vi "modbus slave new.vi"() -> ()   [LabVIEW 2016]
uses:
  <vilib>/NI/Modbus Library/API/Wrapper/Create TCP Slave.vi
  <vilib>/NI/Modbus Library/API/Slave/Modbus Slave.lvclass
  <vilib>/NI/Modbus Library/API/Wrapper/API Main.lvlib
  <vilib>/ptbypt/NI_PtbyPt.lvlib
panel:
  out "status":bool
  in  "写入registers to write":u16[](array[numeric])
  out "读取register values":u16[](array[numeric])
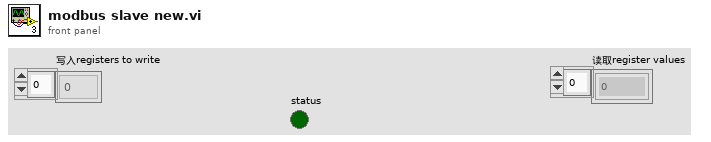
[diagram p1: front panel]
types:
  T1 = cluster{"测量量程":dbl, "测量精度":dbl, "测量间隔":dbl, "消解温度":dbl, "消解时长":dbl, "空白校准时间":timestamp, "曲线截距":dbl, "曲线斜率":dbl, "测量检出限":dbl, "测量信号值":dbl, "线性相关系数":dbl, "二次多项式系数":dbl, "标样校准时间":timestamp, "单位":u16}
  T2 = typedef "LVDateTimeRec.ctl" = cluster{"秒数的小数部分":dbl, "秒":i32, "分":i32, "时":i32, "日":i32, "月":i32, "年":i32, "天数（周）":i32, "天数（年）":i32, "DST":i32}
  T3 = enum16{"启动整机", "停止整机", "标样核查", "加标回收", "平行样测试", "零点核查", "跨度核查", "校零", "校标"}
  T4 = cluster{"status":bool, "代码":u16, "source":string}
  T5 = cluster{"系统时间":timestamp, "工作状态":enum16{"空闲", "水样测试", "标样核查", "零点核查", "跨度核查", "空白测试", "平行样测试", "加标回收", "空白校准", "标样校准", "初始化（清洗）"}, "测量模式":enum16{"待机", "连续模式", "周期模式", "定点模式", "受控模式", "手动模式"}, "告警代码":enum16{"无告警", "缺试剂告警", "缺水样告警", "缺蒸馏水告警", "缺标液告警", "仪表漏液告警", "标定异常告警", "超量程告警", "加热异常", "低试剂预警", "超上限告警", "超下限告警", "仪表内部其他异常", "滴定异常告警", "电极异常告警", "量程切换告警", "参数设置告警", "PH电极电位异常", "电导率电极异常", "浊度光度异常", "溶解氧电极异常", "溶解氧光强异常", "温度异常告警", "PH异常告警", "溶解氧异常告警", "电导率异常告警", "浊度异常告警", "叶绿素异常告警", "藻密度异常告警", "蓝绿藻异常告警", "ORP异常告警", "氨氮异常告警", "清洁刷异常告警", "SD卡异常告警", "蓝牙异常告警", "Wifi异常告警", "流程异常告警"}, "故障代码":enum16{"无故障", "电机故障", "温度故障", "通讯故障", "滴定故障"}, "日志代码":u16, "软件版本":u16, "F0":sgl, "F1":sgl, "F2":sgl, "F3":sgl, "T":sgl, "H":sgl, "id":u16, "flowid":u16, "量程":u16, "总磷控温温度1":sgl, "营养盐控温温度2":sgl, "ADC":sgl}
  T6 = enum16{"空闲", "水样测试", "标样核查", "零点核查", "跨度核查", "空白测试", "平行样测试", "质控样", "空白校准", "标样校准", "加标回收"}
  T7 = enum16{"空闲", "水样测试", "标样核查", "零点核查", "跨度核查", "空白测试", "平行样测试", "加标回收", "空白校准", "标样校准", "初始化（清洗）"}
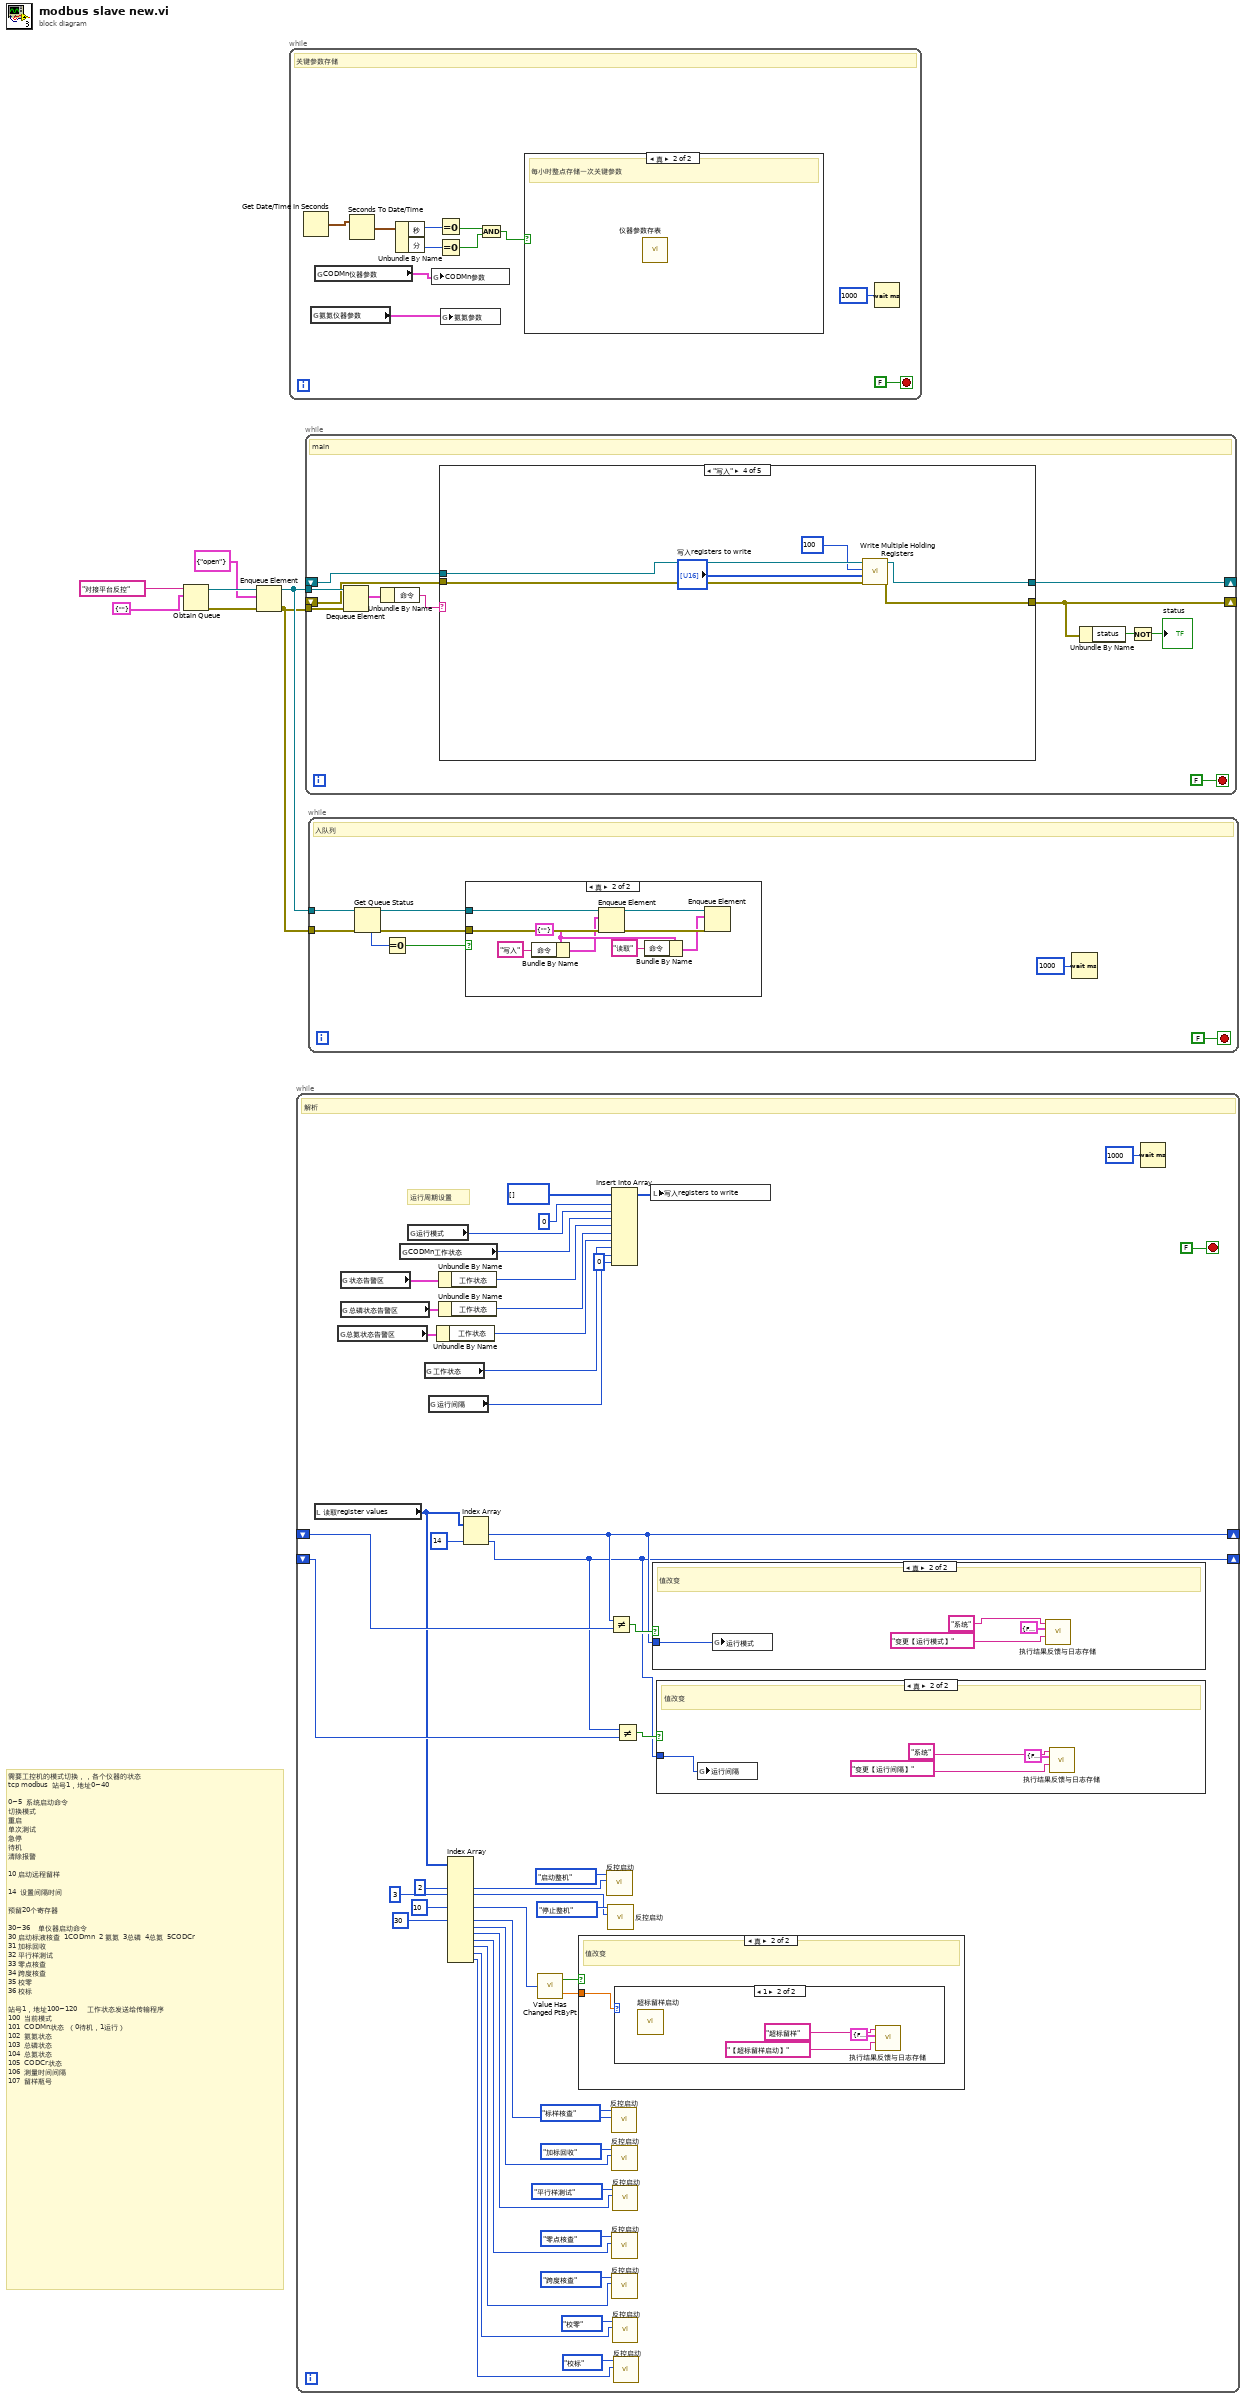
[diagram p0: block diagram]
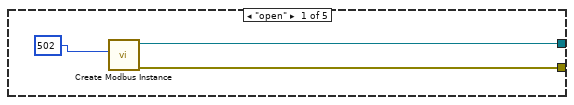
[diagram p8: hidden frame]
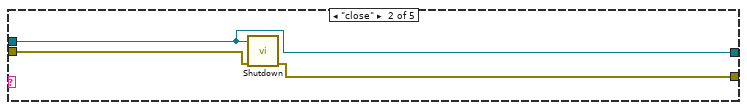
[diagram p9: hidden frame]
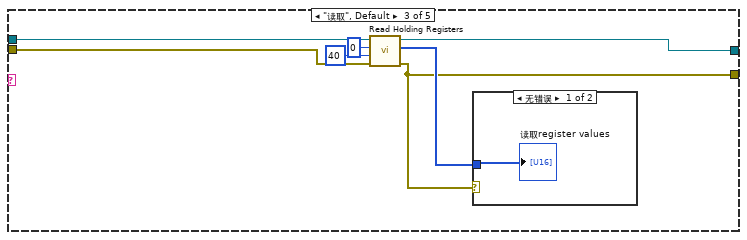
[diagram p10: hidden frame]
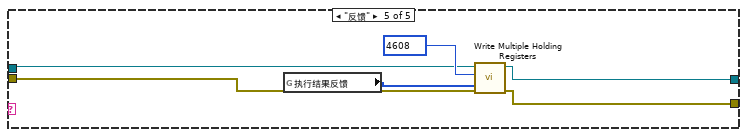
[diagram p12: hidden frame]
diagram:
  # "需要工控机的模式切换，，各个仪器的状态\ntcp modbus  站号1，地址0~40\n\n0~5  系统启动命令\n切换模式\n重启\n单次测试\n急停\n待机\n清除报警\n\n10 启动远程留样\n\n14  设置间隔时间\n\n预留20个寄存器\n\n30~36    单仪器启动命令\n30 启动标液核查  1CODmn  2 氨氮  3总磷  4总氮  5CODCr\n31 加标回收\n32 平行样测试\n33 零点核查\n34 跨度核查\n35 校零\n36 校标\n\n站号1，地址100~120     工作状态发送给传输程序\n100  当前模式\n101  CODMn状态  （0待机，1运行）\n102  氨氮状态\n103  总磷状态\n104  总氮状态\n105  CODCr状态\n106  测量时间间隔\n107  留样瓶号"
  n1 = Obtain Queue(name (unnamed)="对接平台反控" ("名称（未命名）"), element data type=cluster{"命令":string} {"命令"=""}) -> (queue out=w5:refnum<queue>, error out=w4:errorcluster)  [unwired: 3 in, 1 out]
  n2 = Enqueue Element(queue=w5, element=cluster{"命令":string} {"命令"="open"} ("元素"), error in (no error)=w4) -> (queue out=w2:refnum<queue>, error out=w1:errorcluster)  [unwired: 1 in, 1 out]
  n3 = while {
    stop <- FALSE stop-if-true
    # "关键参数存储"
    n4 = Get Date/Time In Seconds() -> (seconds since 1Jan1904=w16:timestamp)
    n5 = global read "氨氮断电保存全局变量.vi" "氨氮仪器参数"() -> (w8:T1)
    n6 = global read "CODMn断电保存全局变量.vi" "CODMn仪器参数"() -> (w9:T1)
    n7 = Seconds To Date/Time(time stamp (now)=w16) -> (date time rec=w15:T2)  [unwired: 1 in]
    n8 = Unbundle By Name(w15) -> ("秒"=w14:i32, "分"=w13:i32)
    n9 = global write "在线监测仪器仪表参数.vi" "CODMn参数"(w9) -> ()
    n10 = Equal To 0?(x=w14) -> (x = 0?=w12:bool)
    n11 = Equal To 0?(x=w13) -> (x = 0?=w11:bool)
    n12 = global write "在线监测仪器仪表参数.vi" "氨氮参数"(w8) -> ()
    n13 = And(x=w12, y=w11) -> (x .and. y?=w10:bool)
    n14 = case shown="真" w10 {
      frame False {
      }
      frame True {
        # "每小时整点存储一次关键参数"
        n15 = call "仪器参数存表.vi"() -> ()  [unwired: 12 in]
      }
    }
    n16 = Wait (ms)(milliseconds to wait=u32 1000 ("等待时间（毫秒）")) -> ()  [unwired: 1 out]
  }
  n17 = while {
    shift-right: [w49] -> _
    shift-left: _ -> [w51]
    shift-right: [w46] -> _
    shift-left: _ -> [w48]
    stop <- FALSE stop-if-true
    # "运行周期设置"
    # "解析"
    n18 = local read "读取register values"() -> (w41:u16[])
    n19 = global read "VAR总磷总氮全局变量.vi" "总氮状态告警区"() -> (w58:T5)
    n20 = global read "VAR氨氮全局变量.vi" "状态告警区"() -> (w62:T5)
    n21 = global read "VAR总磷总氮全局变量.vi" "总磷状态告警区"() -> (w60:T5)
    n22 = global read "COD测量模式全局.vi" "CODMn工作状态"() -> (w56:T6)
    n23 = global read "系统设置全局变量.vi" "运行模式"() -> (w64:enum16{"维护模式", "常规模式", "应急模式", "质控模式"})
    n24 = global read "CODcr全局变量.vi" "工作状态"() -> (w55:T7)
    n25 = global read "系统设置全局变量.vi" "运行间隔"() -> (w54:i16)
    n26 = Unbundle By Name(w58) -> ("工作状态"=w57:T7)
    n27 = Unbundle By Name(w62) -> ("工作状态"=w61:T7)
    n28 = Unbundle By Name(w60) -> ("工作状态"=w59:T7)
    n29 = Index Array(array=w41, index #3=2 ("索引"), index #4=3 ("索引"), index #6=10 ("索引"), index #8=30 ("索引")) -> (element #3=w40:u16, element #4=w37:u16, element #6=w34:u16, element #8=w32:u16, element #9=w26:u16, element #10=w25:u16, element #11=w24:u16, element #12=w22:u16, element #13=w21:u16, element #14=w20:u16)  [unwired: 10 in, 4 out]
    n30 = Index Array(array=w41, index #2=14 ("索引")) -> (element #1=w49:u16, element #2=w46:u16)  [unwired: 1 in]
    n31 = call <vilib>:"Value Has Changed PtByPt.vi"("input data point"=w34) -> ("has changed"=w36:bool, "output data point"=w35:dbl)  [unwired: 1 in]
    n32 = case shown="真" w36 {
      tunnel: w35 -> [_ w68]
      frame False {
      }
      frame True {
        # "值改变"
        n33 = case shown="1" w68 {
          frame 0, Default {
          }
          frame 1 {
            n34 = call "超标留样启动.vi"() -> ()  [unwired: 11 in, 1 out]
            n35 = call "执行结果反馈与日志存储.vi"("日志信息"="【超标留样启动】", "error out"=T4 {"status"=FALSE, "代码"=1, "source"=""}, "设备"="超标留样") -> ()  [unwired: 9 in]
          }
        }
      }
    }
    n36 = call "反控启动.vi"("启动参数"=w40, "启动类型"=T3."启动整机") -> ()  [unwired: 10 in]
    n37 = call "反控启动.vi"("启动参数"=w37, "启动类型"=T3."停止整机") -> ()  [unwired: 10 in]
    n38 = Not Equal?(x=w49, y=w51) -> (x != y?=w50:bool)
    n39 = call "反控启动.vi"("启动参数"=w32, "启动类型"=T3."标样核查") -> ()  [unwired: 10 in]
    n40 = Insert Into Array(array=u16[] [] ("values to write"), index=0 ("索引"), new element #1=w64, new element #2=w56, new element #3=w61, new element #4=w59, new element #5=w57, new element #6=w55, new element #7=w54, new element #8=u16 0 ("新元素/子数组")) -> (w53:u16[])
    n41 = call "反控启动.vi"("启动参数"=w26, "启动类型"=T3."加标回收") -> ()  [unwired: 10 in]
    n42 = call "反控启动.vi"("启动参数"=w24, "启动类型"=T3."零点核查") -> ()  [unwired: 10 in]
    n43 = call "反控启动.vi"("启动参数"=w22, "启动类型"=T3."跨度核查") -> ()  [unwired: 10 in]
    n44 = call "反控启动.vi"("启动参数"=w25, "启动类型"=T3."平行样测试") -> ()  [unwired: 10 in]
    n45 = call "反控启动.vi"("启动参数"=w21, "启动类型"=T3."校零") -> ()  [unwired: 10 in]
    n46 = call "反控启动.vi"("启动参数"=w20, "启动类型"=T3."校标") -> ()  [unwired: 10 in]
    n47 = Not Equal?(x=w46, y=w48) -> (x != y?=w47:bool)
    n48 = local write "写入registers to write"(w53) -> ()
    n49 = case shown="真" w50 {
      tunnel: w49 -> [_ w79]
      frame False {
      }
      frame True {
        # "值改变"
        n50 = global write "系统设置全局变量.vi" "运行模式"(w79) -> ()
        n51 = call "执行结果反馈与日志存储.vi"("日志信息"="变更【运行模式】", "error out"=T4 {"status"=FALSE, "代码"=1, "source"=""}, "设备"="系统") -> ()  [unwired: 9 in]
      }
    }
    n52 = case shown="真" w47 {
      tunnel: w46 -> [_ w75]
      frame False {
      }
      frame True {
        # "值改变"
        n53 = global write "系统设置全局变量.vi" "运行间隔"(w75) -> ()
        n54 = call "执行结果反馈与日志存储.vi"("日志信息"="变更【运行间隔】", "error out"=T4 {"status"=FALSE, "代码"=1, "source"=""}, "设备"="系统") -> ()  [unwired: 9 in]
      }
    }
    n55 = Wait (ms)(milliseconds to wait=u32 1000 ("等待时间（毫秒）")) -> ()  [unwired: 1 out]
  }
  n56 = while {
    tunnel: w2 -> [w90]
    tunnel: w1 -> [w89]
    shift-right: [w86] -> _
    shift-left: _ -> [w85]
    shift-right: [w80] -> _
    shift-left: _ -> [w84]
    stop <- FALSE stop-if-true
    # "main"
    n57 = Dequeue Element(queue=w90, error in (no error)=w89) -> (element=w88:cluster{"命令":string})  [unwired: 1 in, 3 out]
    n58 = Unbundle By Name(w88) -> ("命令"=w87:string)
    n59 = case shown="\"写入\"" w87 {
      tunnel: [w91 w94 w98 w106 w113] -> w86
      tunnel: [w92 w95 w97 w105 w112] -> w80
      tunnel: w85 -> [_ w94 w103 w110 w115]
      tunnel: w84 -> [_ w96 w102 w109 w114]
      frame "open" {
        n60 = call-poly <vilib>:"Create Modbus Instance.vi"("port (502)"=u16 502) -> ("error out"=w92:errorcluster, "TCP slave instance"=w91:refnum<class "Modbus Slave.lvclass">)  [unwired: 9 in]
      }
      frame "close" {
        n61 = call-dynamic "Shutdown.vi"("error in"=w96, "Modbus slave in"=w94) -> ("error out"=w95:errorcluster)  [unwired: 9 in]
      }
      frame "读取", Default {
        n62 = call-dynamic "Read Holding Registers.vi"("error in"=w102, "number of inputs"=u16 40, "starting address"=u16 0, "Modbus slave in"=w103) -> ("error out"=w97:errorcluster, "register values"=w99:u16[], "Modbus slave out"=w98:refnum<class "Modbus Slave.lvclass">)  [unwired: 5 in]
        n63 = case shown="无错误" w97 {
          tunnel: w99 -> [w104 _]
          frame No Error {
            "读取register values" <- w104
          }
          frame Error {
          }
        }
      }
      frame "写入" {
        n64 = call-dynamic "Write Multiple Holding Registers.vi"("error in"=w109, "registers to write"="写入registers to write", "starting address"=u16 100, "Modbus slave in"=w110) -> ("error out"=w105:errorcluster, "Modbus slave out"=w106:refnum<class "Modbus Slave.lvclass">)  [unwired: 6 in]
      }
      frame "反馈" {
        n65 = global read "modbus slave全局.vi" "执行结果反馈"() -> (w111:u16[])
        n66 = call-dynamic "Write Multiple Holding Registers.vi"("error in"=w114, "registers to write"=w111, "starting address"=u16 4608, "Modbus slave in"=w115) -> ("error out"=w112:errorcluster, "Modbus slave out"=w113:refnum<class "Modbus Slave.lvclass">)  [unwired: 6 in]
      }
    }
    n67 = Unbundle By Name(w80) -> ("status"=w82:bool)
    n68 = Not(x=w82) -> (.not. x?=→"status":bool)
  }
  n69 = while {
    tunnel: w2 -> [w124]
    tunnel: w1 -> [w122]
    stop <- FALSE stop-if-true
    # "入队列"
    n70 = Get Queue Status(queue=w124, error in (no error)=w122) -> (queue out=w123:refnum<queue>, error out=w121:errorcluster, # elements in queue=w120:i32)  [unwired: 1 in, 5 out]
    n71 = Equal To 0?(x=w120) -> (x = 0?=w119:bool)
    n72 = case shown="真" w119 {
      tunnel: w123 -> [_ w133]
      tunnel: w121 -> [_ w132]
      frame False {
      }
      frame True {
        w128 = cluster{"命令":string} {"命令"=""} ("元素")
        n73 = Bundle By Name(cluster=w128, "命令"="写入") -> (w127:cluster{"命令":string})
        n74 = Enqueue Element(queue=w133, element=w127, error in (no error)=w132) -> (queue out=w131:refnum<queue>, error out=w130:errorcluster)  [unwired: 1 in, 1 out]
        n75 = Bundle By Name(cluster=w128, "命令"="读取") -> (w125:cluster{"命令":string})
        n76 = Enqueue Element(queue=w131, element=w125, error in (no error)=w130) -> ()  [unwired: 1 in, 3 out]
      }
    }
    n77 = Wait (ms)(milliseconds to wait=u32 1000 ("等待时间（毫秒）")) -> ()  [unwired: 1 out]
  }
